vi "FlatToRichcif_manager_FileData.vi"(5 "OutputClusterType":T1, 11 "InputCluster":T2) -> (3 "OutputCluster":T1)   [LabVIEW 2021, in "CIF_Launcher_client.lvlib"]
uses:
  CIF_Launcher_client.lvlib
  cif_manager_FileData_Flat.ctl
  cif_manager_FileData.ctl
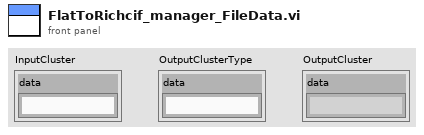
[diagram p1: front panel]
types:
  T1 = typedef "CIF_Launcher_client.lvlib/cif_manager_FileData.ctl" = cluster{"data":string}
  T2 = typedef "CIF_Launcher_client.lvlib/cif_manager_FileData_Flat.ctl" = cluster{"data":string}
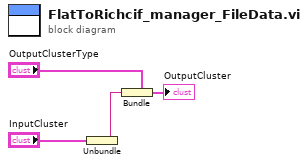
[diagram p0: block diagram]
diagram:
  n1 = Unbundle "Unbundle"("InputCluster") -> ("data"=w1:string)
  n2 = Bundle "Bundle"(cluster="OutputClusterType", "data"=w1) -> (→"OutputCluster":T1)
